vi "BL_GetData.vi"(8 "error in (no error)":errorcluster, 10 "Channel":u8, 11 "Potentiostat Galvanostat in":refnum<class "Potentiostat Galvanostat.lvclass">) -> (0 "error out":errorcluster, 1 "Data Buffer":u32[][](array[numeric]), 2 "Channel":u8, 3 "Potentiostat Galvanostat out":refnum<class "Potentiostat Galvanostat.lvclass">, 5 "Current Values":T1 {"State" items=["Channel is stopped", "Channel is running", "Channel is paused"]; "I Range" items=["I range 100 pA SP-300 series", "I range 1 nA VMP3 / SP-300 series", "I range 10 nA VMP3 / SP-300 series", "I range 100 nA VMP3 / SP-300 series", "I range 1 uA VMP3 / SP-300 series", "I range 10 uA VMP3 / SP-300 series", "I range 100 uA VMP3 / SP-300 series", "I range 1 mA VMP3 / SP-300 series", "I range 10 mA VMP3 / SP-300 series", "I range 100 mA VMP3 / SP-300 series", "I range 1 A VMP3 / SP-300 series", "Booster VMP3 / SP-300 series", "Auto range VMP3 / SP-300 series"]; "Hardware Option Error Code" items=["No Error"=0, "no instrument connected"=-1, "connection in progress"=-2, "selected channel(s) unplugged"=-3, "invalid function parameters"=-4, "selected file does not exist"=-5, "function failed"=-6, "no channel selected"=-7, "invalid instrument configuration"=-8, "EC-Lab firmware loaded on the instrument"=-9, "library not correctly loaded in memory"=-10, "USB library not correctly loaded in memory"=-11, "function of the library already in progress"=-12, "selected channel(s) already used"=-13, "device not allowed"=-14, "Invalid update function parameters"=-15, "internal instrument communication failed"=-101, "too many data to transfer from the instrument (device error)"=-102, "selected channel(s) unplugged (device error)"=-103, "instrument response error"=-104, "invalid message size"=-105]}, 7 "Data Information":T5)   [LabVIEW 2018, in "Potentiostat Galvanostat.lvclass"]
doc: "The hardware conf object. The attribute “Conn” is the electrode\nconnection mode and the attribute “Ground” is the instrument\nground. See 5. Structures and Constants to have the value of these\nattributes."
uses:
  Potentiostat Galvanostat.lvclass
  Controls/Data Information.ctl
  Controls/Technique ID.ctl
  Controls/Current Values.ctl
  Controls/Channel State.ctl
  Controls/Current Range.ctl
  Controls/Error Codes.ctl
  Potentiostat Galvanostat.lvclass/Potentiostat Galvanostat.ctl
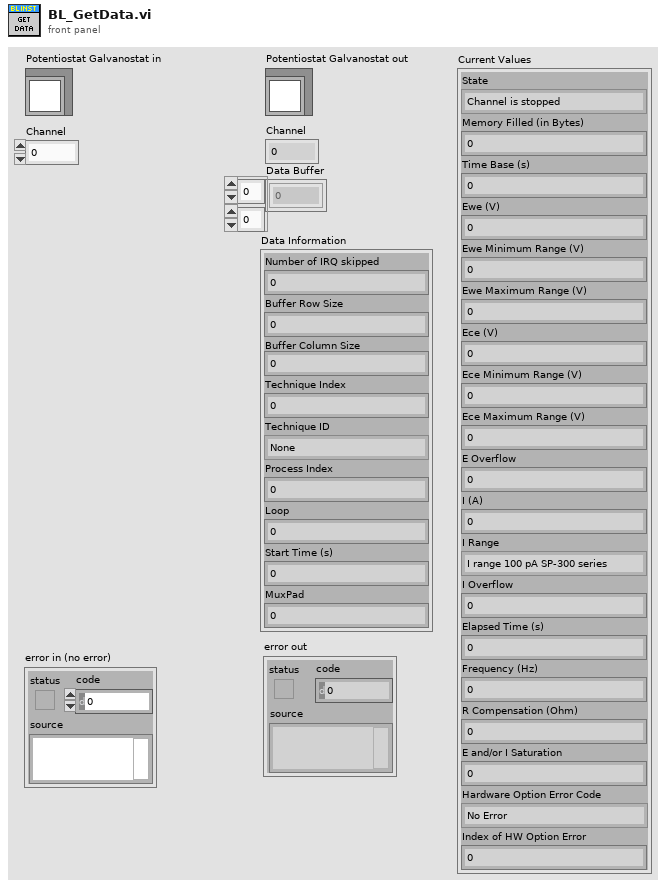
[diagram p1: front panel]
types:
  T1 = typedef "Potentiostat Galvanostat.lvclass/Current Values.ctl" = cluster{"State":T2, "Memory Filled (in Bytes)":i32, "Time Base (s)":sgl, "Ewe (V)":sgl, "Ewe Minimum Range (V)":sgl, "Ewe Maximum Range (V)":sgl, "Ece (V)":sgl, "Ece Minimum Range (V)":sgl, "Ece Maximum Range (V)":sgl, "E Overflow":i32, "I (A)":sgl, "I Range":T3, "I Overflow":i32, "Elapsed Time (s)":dbl, "Frequency (Hz)":sgl, "R Compensation (Ohm)":sgl, "E and/or I Saturation":sgl, "Hardware Option Error Code":T4, "Index of HW Option Error":i32}
  T2 = typedef "Potentiostat Galvanostat.lvclass/Channel State.ctl" = i32
  T3 = typedef "Potentiostat Galvanostat.lvclass/Current Range.ctl" = i32
  T4 = typedef "Potentiostat Galvanostat.lvclass/Error Codes.ctl" = i32
  T5 = typedef "Potentiostat Galvanostat.lvclass/Data Information.ctl" = cluster{"Number of IRQ skipped":i32, "Buffer Row Size":i32, "Buffer Column Size":i32, "Technique Index":i32, "Technique ID":T6, "Process Index":i32, "Loop":i32, "Start Time (s)":sgl, "MuxPad":i32}
  T6 = typedef "Potentiostat Galvanostat.lvclass/Technique ID.ctl" = i32
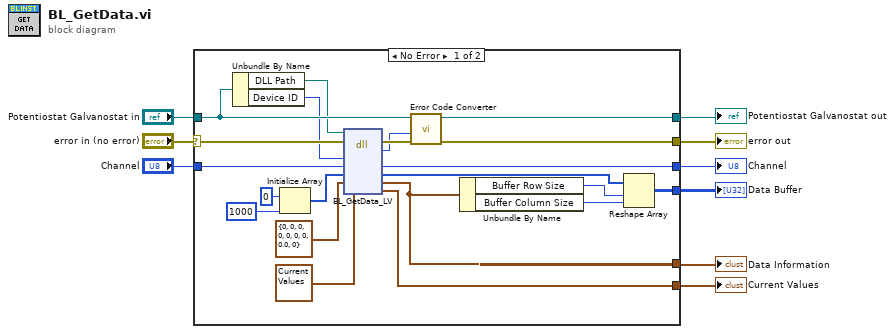
[diagram p0: block diagram]
diagram:
  n1 = case shown="No Error" "error in (no error)" {
    selector: "error in (no error)" -> [w22 w32]
    tunnel: [w30 w32] -> w8
    tunnel: [w29 w31] -> w6
    tunnel: "Potentiostat Galvanostat in" -> [w28 w31]
    tunnel: "Channel" -> [w18 _]
    tunnel: [w17 _] -> w4
    tunnel: [w13 _] -> w2
    tunnel: [w15 _] -> w3
    tunnel: [w10 _] -> w1
    frame No Error {
      n2 = Unbundle By Name(w28) -> ("DLL Path"=w19:path, "Device ID"=w20:i32)
      n3 = Initialize Array(u32 0, 1000 ("dimension size")) -> (w27:u32[])
      n4 = dll-call lib="C:/Projects/LabVIEW/BioLogic Instrument Driver/libs/EC-Lab Development Package/EClib.dll" fn="BL_GetData_LV"(path in=w19, error in=w22, "Device ID"=w20, "Channel"=w18, "Data Buffer"=w27, "Data Information"=T5 {"Number of IRQ skipped"=0, "Buffer Row Size"=0, "Buffer Column Size"=0, "Technique Index"=0, "Technique ID"=0, "Process Index"=0, "Loop"=0, "Start Time (s)"=0.0, "MuxPad"=0}, "Current Values"=T1 {"State"=0, "Memory Filled (in Bytes)"=0, "Time Base (s)"=0.0, "Ewe (V)"=0.0, "Ewe Minimum Range (V)"=0.0, "Ewe Maximum Range (V)"=0.0, "Ece (V)"=0.0, "Ece Minimum Range (V)"=0.0, "Ece Maximum Range (V)"=0.0, "E Overflow"=0, "I (A)"=0.0, "I Range"=0, "I Overflow"=0, "Elapsed Time (s)"=0.0, "Frequency (Hz)"=0.0, "R Compensation (Ohm)"=0.0, "E and/or I Saturation"=0.0, "Hardware Option Error Code"=0, "Index of HW Option Error"=0}) -> (error out=w21:errorcluster, "Error Code"=w16:i32, "Channel"=w17:u8, "Data Buffer"=w14:u32[], "Data Information"=w13:T5, "Current Values"=w15:T1)  [unwired: 2 in, 1 out]
      n5 = call-dynamic "Error Code Converter.vi"("error in (no error)"=w21, "Error Code"=w16, "Potentiostat Galvanostat in"=w28) -> ("error out"=w30:errorcluster, "Potentiostat Galvanostat out"=w29:refnum<class "Potentiostat Galvanostat.lvclass">)  [unwired: 7 in]
      n6 = Unbundle By Name(w13) -> ("Buffer Row Size"=w12:i32, "Buffer Column Size"=w11:i32)
      n7 = Reshape Array(w14, w12, w11) -> (w10:u32[][])
    }
    frame Error {
    }
  }
  "error out" <- w8
  "Potentiostat Galvanostat out" <- w6
  "Channel" <- w4
  "Data Information" <- w2
  "Current Values" <- w3
  "Data Buffer" <- w1
